vi "test_Rx Exec Unit (UDP).vi"() -> ()   [LabVIEW 2020]
uses:
  <vilib>/NI VeriStand/Custom Device API/Custom Device Item Ref.ctl
  <vilib>/NI VeriStand/Custom Device API/Custom Device API.lvlib
  Engine/Implementation/Rx UDP Execution Unit/Rx UDP Execution Unit.lvclass
  Engine/Implementation/Shared Resources/Shared Resources.lvclass
  C:/Users/Administrator/Desktop/git/niveristand-aim-arinc664-custom-device/Source/Custom Device Support/Engine/Interfaces/Shared Resources/Shared Resources.lvclass
  <instrlib>/AIM GmbH/_AIM 664/_controls/comm_verification_rx.ctl
  <instrlib>/AIM GmbH/_AIM 664/AIM664LV.lvlib
  Import/_typedefs/board_setup.ctl
  Import/AIM ARINC 664 Import.lvlib
  Shared/Encoding (Arinc664).ctl
  <instrlib>/AIM GmbH/_AIM 664/_controls/comm_udp_rx.ctl
panel:
  in  "board properties in":T1={"boardId"=1, "portSpeed"=0, "portConfig"=0} {"portConfig" items=["FDX_SINGLE", "FDX_REDUNDANT"]; "portSpeed" items=["FDX_100MBIT", "FDX_10MBIT", "FDX_AUTO_100MBIT", "FDX_AUTO_10MBIT", "FDX_AUTO_ERROR", "FDX_1000MBIT"]}
  in  "Init Shared Resources":bool
  in  "rx_param":T3(array[cluster])=[{"Data"=[0, 0, 0, 0, 0, 0, 0, 0, 0, 0, 0, 0, 0, 0, 0, 0, 0, 0, 0, 0, 0, 0, 0, 0, 0, 0, 0, 0, 0, 0, 0, 0, 0, 0, 0, 0, 0, 0, 0, 0, 0, 0, 0, 0, 0, 0, 0, 0, 0, 0, 0, 0, 0, 0, 0, 0, 0, 0, 0, 0, 0, 0, 0, 0, 0, 0, 0, 0, 0, 0, 0, 0, 0, 0, 0, 0, 0, 0, 0, 0, 0, 0, 0, 0, 0, 0, 0, 0, 0, 0, 0, 0, 0, 0, 0, 0, 0, 0, 0, 0, 0, 0, 0, 0, 0, 0, 0, 0, 0, 0, 0, 0, 0, 0, 0, 0, 0, 0, 0, 0, 0, 0, 0, 0, 0, 0, 0, 0, 0, 0, 0, 0, 0, 0, 0, 0, 0, 0, 0, 0, 0, 0, 0, 0, 0, 0, 0, 0, 0, 0, 0, 0, 0, 0, 0, 0, 0, 0, 0, 0, 0, 0, 0, 0, 0, 0, 0, 0, 0, 0, 0, 0, 0, 0, 0, 0, 0, 0, 0, 0, 0, 0, 0, 0, 0, 0, 0, 0, 0, 0, 0, 0, 0, 0, 0, 0, 0, 0, 0, 0, 0, 0, 0, 0, 0, 0, 0, 0, 0, 0, 0, 0, 0, 0, 0, 0, 0, 0, 0, 0, 0, 0, 0, 0, 0, 0, 0, 0, 0, 0, 0, 0, 0, 0, 0, 0, 0, 0, 0, 0, 0, 0, 0, 0, 0, 0, 0, 0, 0, 0, 0, 0, 0, 0, 0, 0, 0, 0, 0, 0, 0, 0, 0, 0, 0, 0, 0, 0, 0, 0, 0, 0, 0, 0, 0, 0, 0, 0, 0, 0, 0, 0, 0, 0, 0, 0, 0, 0, 0, 0, 0, 0, 0, 0, 0, 0, 0, 0, 0, 0, 0, 0, 0, 0, 0, 0, 0, 0, 0, 0, 0, 0, 0, 0, 0, 0, 0, 0, 0, 0, 0, 0, 0, 0, 0, 0, 0, 0, 0, 0, 0, 0, 0, 0, 0, 0, 0, 0, 0, 0, 0, 0, 0, 0, 0, 0, 0, 0, 0, 0, 0, 0, 0, 0, 0, 0, 0, 0, 0, 0, 0, 0, 0, 0, 0, 0, 0, 0, 0, 0, 0, 0, 0, 0, 0, 0, 0, 0, 0, 0, 0, 0, 0, 0, 0, 0, 0, 0, 0, 0, 0, 0, 0, 0, 0, 0, 0, 0, 0, 0, 0, 0, 0, 0, 0, 0, 0, 0, 0, 0, 0, 0, 0, 0, 0, 0, 0, 0, 0, 0, 0, 0, 0, 0, 0, 0, 0, 0, 0, 0, 0, 0, 0, 0, 0, 0, 0, 0, 0, 0, 0, 0, 0, 0, 0, 0, 0, 0, 0, 0, 0, 0, 0, 0, 0, 0, 0, 0, 0, 0, 0, 0, 0, 0, 0, 0, 0, 0, 0, 0, 0, 0, 0, 0, 0, 0, 0, 0, 0, 0, 0, 0, 0, 0, 0, 0, 0, 0, 0, 0, 0, 0, 0, 0, 0, 0, 0, 0, 0, 0, 0, 0, 0, 0, 0, 0, 0, 0, 0, 0, 0, 0, 0, 0, 0, 0, 0, 0, 0, 0, 0, 0, 0, 0, 0, 0, 0, 0, 0, 0, 0, 0, 0, 0, 0, 0, 0, 0, 0, 0, 0, 0, 0, 0, 0, 0, 0, 0, 0, 0, 0, 0, 0, 0, 0, 0, 0, 0, 0, 0, 0, 0, 0, 0, 0, 0, 0, 0, 0, 0, 0, 0, 0, 0, 0, 0, 0, 0, 0, 0, 0, 0, 0, 0, 0, 0, 0, 0, 0, 0, 0, 0, 0, 0, 0, 0, 0, 0, 0, 0, 0, 0, 0, 0, 0, 0, 0, 0, 0, 0, 0, 0, 0, 0, 0, 0, 0, 0, 0, 0, 0, 0, 0, 0, 0, 0, 0, 0, 0, 0, 0, 0, 0, 0, 0, 0, 0, 0, 0, 0, 0, 0, 0, 0, 0, 0, 0, 0, 0, 0, 0, 0, 0, 0, 0, 0, 0, 0, 0, 0, 0, 0, 0, 0, 0, 0, 0, 0, 0, 0, 0, 0, 0, 0, 0, 0, 0, 0, 0, 0, 0, 0, 0, 0, 0, 0, 0, 0, 0, 0, 0, 0, 0, 0, 0, 0, 0, 0, 0, 0, 0, 0, 0, 0, 0, 0, 0, 0, 0, 0, 0, 0, 0, 0, 0, 0, 0, 0, 0, 0, 0, 0, 0, 0, 0, 0, 0, 0, 0, 0, 0, 0, 0, 0, 0, 0, 0, 0, 0, 0, 0, 0, 0, 0, 0, 0, 0, 0, 0, 0, 0, 0, 0, 0, 0, 0, 0, 0, 0, 0, 0, 0, 0, 0, 0, 0, 0, 0, 0, 0, 0, 0, 0, 0, 0, 0, 0, 0, 0, 0, 0, 0, 0, 0, 0, 0, 0, 0, 0, 0, 0, 0, 0, 0, 0, 0, 0, 0, 0, 0, 0, 0, 0, 0, 0, 0, 0, 0, 0, 0, 0, 0, 0, 0, 0, 0, 0, 0, 0, 0, 0, 0, 0, 0, 0, 0, 0, 0, 0, 0, 0, 0, 0, 0, 0, 0, 0, 0, 0, 0, 0, 0, 0, 0, 0, 0, 0, 0, 0, 0, 0, 0, 0, 0, 0, 0, 0, 0, 0, 0, 0, 0, 0, 0, 0, 0, 0, 0, 0, 0, 0, 0, 0, 0, 0, 0, 0, 0, 0, 0, 0, 0, 0, 0, 0, 0, 0, 0, 0, 0, 0, 0, 0, 0, 0, 0, 0, 0, 0, 0, 0, 0, 0, 0, 0, 0, 0, 0, 0, 0, 0, 0, 0, 0, 0, 0, 0, 0, 0, 0, 0, 0, 0, 0, 0, 0, 0, 0, 0, 0, 0, 0, 0, 0, 0, 0, 0, 0, 0, 0, 0, 0, 0, 0, 0, 0, 0, 0, 0, 0, 0, 0, 0, 0, 0, 0, 0, 0, 0, 0, 0, 0, 0, 0, 0, 0, 0, 0, 0, 0, 0, 0, 0, 0, 0, 0, 0, 0, 0, 0, 0, 0, 0, 0, 0, 0, 0, 0, 0, 0, 0, 0, 0, 0, 0, 0, 0, 0, 0, 0], "Parameters"=[{"start index"=0, "size"=64, "encoding"=6, "signed"=TRUE, "scale multiplier"=1.0, "scale offset"=0.0}, {"start index"=64, "size"=64, "encoding"=6, "signed"=TRUE, "scale multiplier"=1.0, "scale offset"=0.0}, {"start index"=0, "size"=0, "encoding"=0, "signed"=FALSE, "scale multiplier"=0.0, "scale offset"=0.0}]}, {"Data"=[0, 0, 0, 0, 0, 0, 0, 0, 0, 0, 0, 0, 0, 0, 0, 0, 0, 0, 0, 0, 0, 0, 0, 0, 0, 0, 0, 0, 0, 0, 0, 0, 0, 0, 0, 0, 0, 0, 0, 0, 0, 0, 0, 0, 0, 0, 0, 0, 0, 0, 0, 0, 0, 0, 0, 0, 0, 0, 0, 0, 0, 0, 0, 0, 0, 0, 0, 0, 0, 0, 0, 0, 0, 0, 0, 0, 0, 0, 0, 0, 0, 0, 0, 0, 0, 0, 0, 0, 0, 0, 0, 0, 0, 0, 0, 0, 0, 0, 0, 0, 0, 0, 0, 0, 0, 0, 0, 0, 0, 0, 0, 0, 0, 0, 0, 0, 0, 0, 0, 0, 0, 0, 0, 0, 0, 0, 0, 0, 0, 0, 0, 0, 0, 0, 0, 0, 0, 0, 0, 0, 0, 0, 0, 0, 0, 0, 0, 0, 0, 0, 0, 0, 0, 0, 0, 0, 0, 0, 0, 0, 0, 0, 0, 0, 0, 0, 0, 0, 0, 0, 0, 0, 0, 0, 0, 0, 0, 0, 0, 0, 0, 0, 0, 0, 0, 0, 0, 0, 0, 0, 0, 0, 0, 0, 0, 0, 0, 0, 0, 0, 0, 0, 0, 0, 0, 0, 0, 0, 0, 0, 0, 0, 0, 0, 0, 0, 0, 0, 0, 0, 0, 0, 0, 0, 0, 0, 0, 0, 0, 0, 0, 0, 0, 0, 0, 0, 0, 0, 0, 0, 0, 0, 0, 0, 0, 0, 0, 0, 0, 0, 0, 0, 0, 0, 0, 0, 0, 0, 0, 0, 0, 0, 0, 0, 0, 0, 0, 0, 0, 0, 0, 0, 0, 0, 0, 0, 0, 0, 0, 0, 0, 0, 0, 0, 0, 0, 0, 0, 0, 0, 0, 0, 0, 0, 0, 0, 0, 0, 0, 0, 0, 0, 0, 0, 0, 0, 0, 0, 0, 0, 0, 0, 0, 0, 0, 0, 0, 0, 0, 0, 0, 0, 0, 0, 0, 0, 0, 0, 0, 0, 0, 0, 0, 0, 0, 0, 0, 0, 0, 0, 0, 0, 0, 0, 0, 0, 0, 0, 0, 0, 0, 0, 0, 0, 0, 0, 0, 0, 0, 0, 0, 0, 0, 0, 0, 0, 0, 0, 0, 0, 0, 0, 0, 0, 0, 0, 0, 0, 0, 0, 0, 0, 0, 0, 0, 0, 0, 0, 0, 0, 0, 0, 0, 0, 0, 0, 0, 0, 0, 0, 0, 0, 0, 0, 0, 0, 0, 0, 0, 0, 0, 0, 0, 0, 0, 0, 0, 0, 0, 0, 0, 0, 0, 0, 0, 0, 0, 0, 0, 0, 0, 0, 0, 0, 0, 0, 0, 0, 0, 0, 0, 0, 0, 0, 0, 0, 0, 0, 0, 0, 0, 0, 0, 0, 0, 0, 0, 0, 0, 0, 0, 0, 0, 0, 0, 0, 0, 0, 0, 0, 0, 0, 0, 0, 0, 0, 0, 0, 0, 0, 0, 0, 0, 0, 0, 0, 0, 0, 0, 0, 0, 0, 0, 0, 0, 0, 0, 0, 0, 0, 0, 0, 0, 0, 0, 0, 0, 0, 0, 0, 0, 0, 0, 0, 0, 0, 0, 0, 0, 0, 0, 0, 0, 0, 0, 0, 0, 0, 0, 0, 0, 0, 0, 0, 0, 0, 0, 0, 0, 0, 0, 0, 0, 0, 0, 0, 0, 0, 0, 0, 0, 0, 0, 0, 0, 0, 0, 0, 0, 0, 0, 0, 0, 0, 0, 0, 0, 0, 0, 0, 0, 0, 0, 0, 0, 0, 0, 0, 0, 0, 0, 0, 0, 0, 0, 0, 0, 0, 0, 0, 0, 0, 0, 0, 0, 0, 0, 0, 0, 0, 0, 0, 0, 0, 0, 0, 0, 0, 0, 0, 0, 0, 0, 0, 0, 0, 0, 0, 0, 0, 0, 0, 0, 0, 0, 0, 0, 0, 0, 0, 0, 0, 0, 0, 0, 0, 0, 0, 0, 0, 0, 0, 0, 0, 0, 0, 0, 0, 0, 0, 0, 0, 0, 0, 0, 0, 0, 0, 0, 0, 0, 0, 0, 0, 0, 0, 0, 0, 0, 0, 0, 0, 0, 0, 0, 0, 0, 0, 0, 0, 0, 0, 0, 0, 0, 0, 0, 0, 0, 0, 0, 0, 0, 0, 0, 0, 0, 0, 0, 0, 0, 0, 0, 0, 0, 0, 0, 0, 0, 0, 0, 0, 0, 0, 0, 0, 0, 0, 0, 0, 0, 0, 0, 0, 0, 0, 0, 0, 0, 0, 0, 0, 0, 0, 0, 0, 0, 0, 0, 0, 0, 0, 0, 0, 0, 0, 0, 0, 0, 0, 0, 0, 0, 0, 0, 0, 0, 0, 0, 0, 0, 0, 0, 0, 0, 0, 0, 0, 0, 0, 0, 0, 0, 0, 0, 0, 0, 0, 0, 0, 0, 0, 0, 0, 0, 0, 0, 0, 0, 0, 0, 0, 0, 0, 0, 0, 0, 0, 0, 0, 0, 0, 0, 0, 0, 0, 0, 0, 0, 0, 0, 0, 0, 0, 0, 0, 0, 0, 0, 0, 0, 0, 0, 0, 0, 0, 0, 0, 0, 0, 0, 0, 0, 0, 0, 0, 0, 0, 0, 0, 0, 0, 0, 0, 0, 0, 0, 0, 0, 0, 0, 0, 0, 0, 0, 0, 0, 0, 0, 0, 0, 0, 0, 0, 0, 0, 0, 0, 0, 0, 0, 0, 0, 0, 0, 0, 0, 0, 0, 0, 0, 0, 0, 0, 0, 0, 0, 0, 0, 0, 0, 0, 0, 0, 0, 0, 0, 0, 0, 0, 0, 0, 0, 0, 0, 0, 0, 0, 0, 0, 0, 0, 0, 0, 0, 0, 0, 0, 0, 0, 0, 0, 0, 0, 0, 0, 0, 0, 0, 0, 0, 0, 0, 0, 0, 0, 0, 0, 0, 0, 0, 0, 0, 0, 0, 0, 0, 0, 0, 0, 0, 0, 0, 0, 0, 0, 0, 0, 0, 0, 0, 0, 0, 0, 0, 0, 0, 0, 0, 0, 0, 0, 0, 0, 0, 0, 0, 0, 0, 0, 0, 0, 0, 0, 0, 0, 0, 0, 0, 0, 0, 0, 0, 0, 0, 0, 0, 0, 0, 0], "Parameters"=[{"start index"=0, "size"=64, "encoding"=6, "signed"=TRUE, "scale multiplier"=1.0, "scale offset"=0.0}, {"start index"=64, "size"=64, "encoding"=6, "signed"=TRUE, "scale multiplier"=1.0, "scale offset"=0.0}, {"start index"=0, "size"=0, "encoding"=0, "signed"=FALSE, "scale multiplier"=0.0, "scale offset"=0.0}]}] {"Parameters"."encoding" items=["BNR", "BCD", "Discrete"]}
  in  "VL Configurations":T6(array[cluster])=[{"VL Config"={"VlId"=60, "VLRange"=1, "VerificationMode"=0, "Bag"=0, "Jitter"=0, "MaxFrameLength"=0, "MaxSkew"=0, "VLBufSize"=32768, "FilterMode"=0, "FilterPosition"=0, "Padding"=0, "FilterMask"=0, "FilterData"=0, "MinFrameLength"=0}, "CommPort Config"=[{"PortType"=enum."FDX_UDP_SAMPLING", "SubVIId"=0, "domainID"=1, "sideID"=1, "locationID"=1, "partitionID"=1, "UdpSrcPort"=24, "UdpDstPort"=23, "UdpNumBufMessages"=1, "UdpMaxMessageSize"=512, "UdpSamplingRate"=0}, {"PortType"=enum."FDX_UDP_SAMPLING", "SubVIId"=0, "domainID"=2, "sideID"=1, "locationID"=1, "partitionID"=1, "UdpSrcPort"=34, "UdpDstPort"=33, "UdpNumBufMessages"=1, "UdpMaxMessageSize"=512, "UdpSamplingRate"=0}]}] {"VL Config"."FilterMode" items=["FDX_RX_VL_FLT_DIS", "FDX_RX_VL_FLT_ENA ", "FDX_RX_VL_FLT_ENA_INV"]; "VL Config"."VLBufSize" format="%.0x"; "VL Config"."VerificationMode" items=["FDX_RX_VL_CHECK_ENA_DEFAULT"=65535, "FDX_RX_VL_CHECK_REDMAM"=16, "DX_RX_VL_CHECK_TRAFIC"=8, "FDX_RX_VL_CHECK_FRAMESIZE"=4, "FDX_RX_VL_CHECK_SNINTEG"=2, "FDX_RX_VL_CHECK_INVPAC"=1, "FDX_RX_VL_CHECK_DISA"=0]}
  in  "port id":u32
  in  "board id":u32=1
  out "exec time us":u32(graph)=2
  out "Values out":dbl[](array[numeric])
  out "error out":errorcluster
  in  "stop":bool
  in  "loop rate mS":u32=10
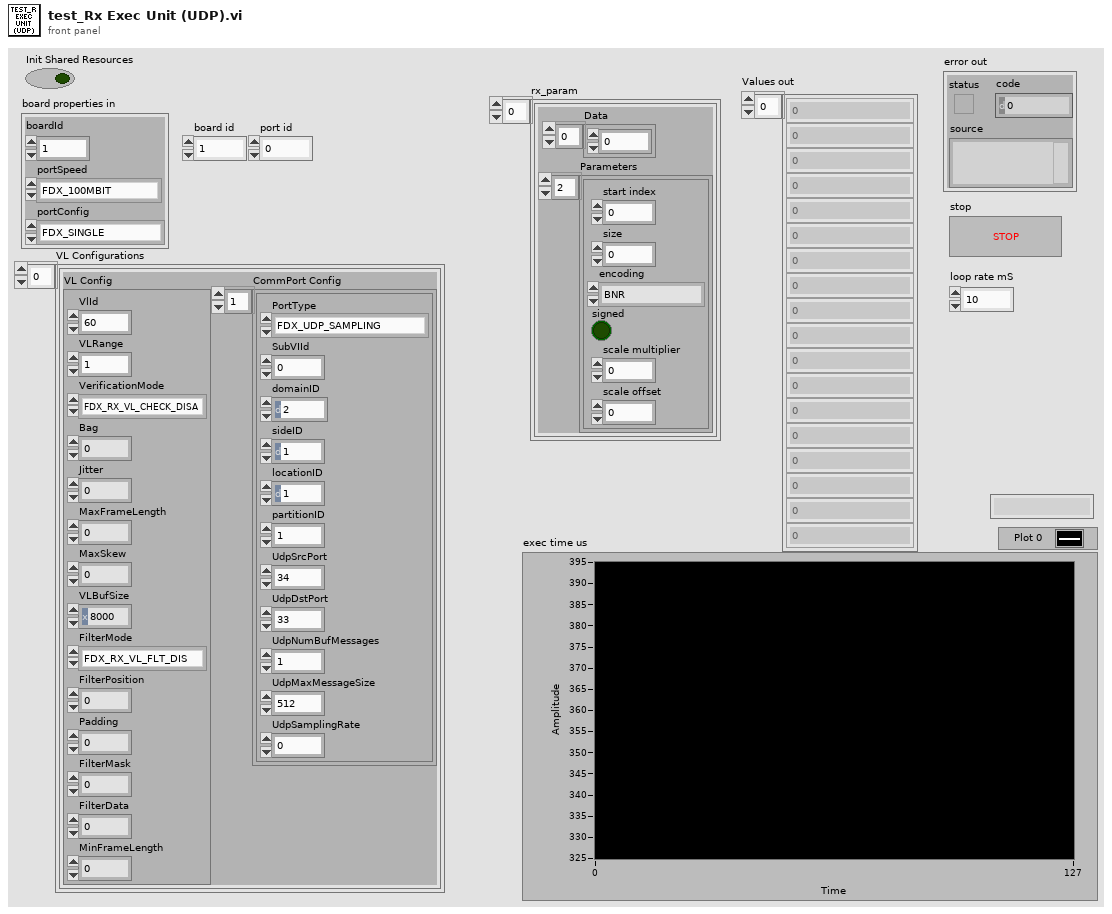
[diagram p1: front panel]
types:
  T1 = typedef "AIM ARINC 664 Import.lvlib/board_setup.ctl" = cluster{"boardId":u32, "portSpeed":u32, "portConfig":u32}
  T2 = typedef "Encoding (Arinc664).ctl" = u16
  T3 = cluster{"Data":u8[], "Parameters":cluster{"start index":i32, "size":i32, "encoding":T2, "signed":bool, "scale multiplier":dbl, "scale offset":dbl}[]}[]
  T4 = typedef "AIM664LV.lvlib/comm_verification_rx.ctl" = cluster{"VlId":u16, "VLRange":u32, "VerificationMode":u32, "Bag":u32, "Jitter":u32, "MaxFrameLength":u32, "MaxSkew":u32, "VLBufSize":u32, "FilterMode":u32, "FilterPosition":u32, "Padding":u32, "FilterMask":u32, "FilterData":u32, "MinFrameLength":u32}
  T5 = typedef "AIM664LV.lvlib/comm_udp_rx.ctl" = cluster{"PortType":enum16{"FDX_UDP_SAMPLING", "FDX_UDP_QUEUING"}, "SubVIId":u32, "domainID":u8, "sideID":u8, "locationID":u8, "partitionID":u8, "UdpSrcPort":u16, "UdpDstPort":u16, "UdpNumBufMessages":u32, "UdpMaxMessageSize":u32, "UdpSamplingRate":u32}
  T6 = cluster{"VL Config":T4, "CommPort Config":T5[]}[]
  T7 = typedef "Custom Device API.lvlib/Custom Device Item Ref.ctl" = u64
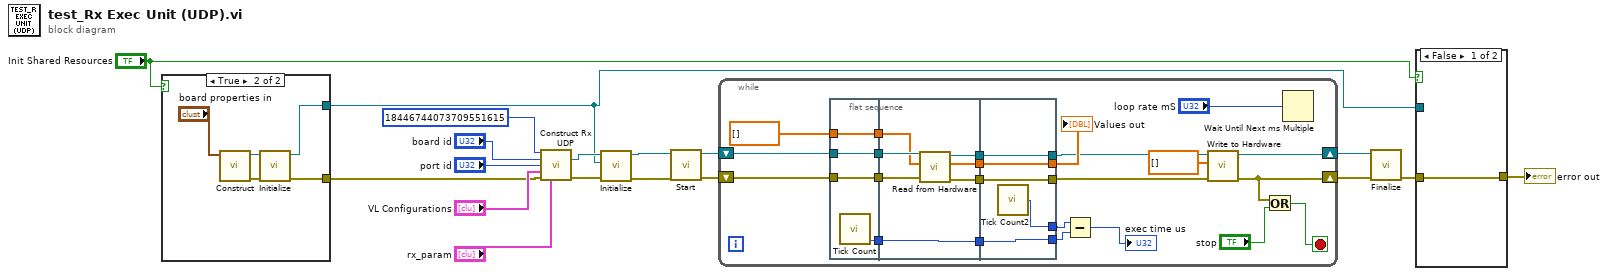
[diagram p0: block diagram]
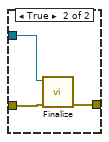
[diagram p2: hidden frame]
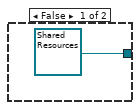
[diagram p3: hidden frame]
diagram:
  n1 = case shown="True" "Init Shared Resources" {
    tunnel: [refnum<class "Shared Resources.lvclass"> refnum ("Shared Resources out") w22] -> w1
    tunnel: [_ w21] -> w5
    frame False {
    }
    frame True {
      n2 = call "Construct.vi"("board properties in"="board properties in") -> ("error out"=w23:errorcluster, "Shared Resources out"=w24:refnum<class "Shared Resources.lvclass">)  [unwired: 9 in]
      n3 = call-dynamic "Initialize.vi"("error in"=w23, "Shared Resources in"=w24) -> ("error out"=w21:errorcluster, "Shared Resources out"=w22:refnum<class "Shared Resources.lvclass">)  [unwired: 8 in]
    }
  }
  n4 = call "Construct Rx UDP.vi"("custom device ref in"=T7 18446744073709551615, "InstrumentHandle_board"="board id", "InstrumentHandle_port"="port id", "VL Configurations"="VL Configurations", "error in (no error)"=w5, "CommPort Payload"="rx_param") -> ("Execution Unit Out"=w11:refnum<class "Rx UDP Execution Unit.lvclass">, "error out"=w12:errorcluster)  [unwired: 7 in, 1 out]
  n5 = call-dynamic "Initialize.vi"("error in"=w12, "shared resources"=w1, "Rx UDP Execution Unit in"=w11) -> ("error out"=w13:errorcluster, "Rx UDP Execution Unit out"=w18:refnum<class "Rx UDP Execution Unit.lvclass">)  [unwired: 7 in]
  n6 = call-dynamic "Start.vi"("error in"=w13, "Rx UDP Execution Unit in"=w18) -> ("error out"=w16:errorcluster, "Rx UDP Execution Unit out"=w17:refnum<class "Rx UDP Execution Unit.lvclass">)  [unwired: 8 in]
  n7 = while {
    shift-right: [w27] -> w15
    shift-left: w17 -> [w47]
    shift-right: [w26] -> w14
    shift-left: w16 -> [w46]
    stop <- w43 stop-if-true
    n8 = flat-sequence {
      tunnel: dbl[] [] ("Values in") -> [w49]
      tunnel: w46 -> [w50]
      tunnel: w47 -> [w51]
      tunnel: [w51] -> w37
      tunnel: [w50] -> w36
      tunnel: [w49] -> w35
      tunnel: [w48] -> w33
      tunnel: [w56] -> w40
      tunnel: [w55] -> w39
      tunnel: [w54] -> w38
      tunnel: w37 -> [w58]
      tunnel: w36 -> [w57]
      tunnel: w35 -> [w53]
      tunnel: [w52] -> w34
      tunnel: w33 -> [w52]
      tunnel: [w61] -> w42
      tunnel: [w62] -> w28
      tunnel: [w63] -> w29
      tunnel: w40 -> [w63]
      tunnel: w39 -> [w62]
      tunnel: w38 -> [w61]
      tunnel: [w60] -> w32
      tunnel: w34 -> [w60]
      tunnel: [w59] -> w31
      frame #0 {
        n9 = call "Tick Count"() -> ("Tick Count(uSec)"=w48:u32)
      }
      frame #1 {
        n10 = call-dynamic "Read from Hardware.vi"("error in"=w57, "Values in"=w53, "Rx UDP Execution Unit in"=w58) -> ("error out"=w55:errorcluster, "Values out"=w54:dbl[], "Rx UDP Execution Unit out"=w56:refnum<class "Rx UDP Execution Unit.lvclass">)  [unwired: 6 in]
      }
      frame #2 {
        n11 = call "Tick Count2"() -> ("Tick Count(uSec)"=w59:u32)
      }
    }
    n12 = Subtract(x=w31, y=w32) -> (x-y=→"exec time us":u32)
    n13 = call-dynamic "Write to Hardware.vi"("error in"=w28, "Values in"=dbl[] [], "Rx UDP Execution Unit in"=w29) -> ("error out"=w26:errorcluster, "Rx UDP Execution Unit out"=w27:refnum<class "Rx UDP Execution Unit.lvclass">)  [unwired: 5 in, 2 out]
    n14 = Or(x=w26, y="stop") -> (x .or. y?=w43:bool)
    n15 = Wait Until Next ms Multiple(millisecond multiple="loop rate mS") -> ()  [unwired: 1 out]
    "Values out" <- w42
  }
  n16 = call-dynamic "Finalize.vi"("error in"=w14, "Rx UDP Execution Unit in"=w15) -> ("error out"=w3:errorcluster)  [unwired: 8 in, 1 out]
  n17 = case shown="False" "Init Shared Resources" {
    tunnel: w3 -> [w64 w66]
    tunnel: [w64 w67] -> w2
    tunnel: w1 -> [_ w65]
    frame False {
    }
    frame True {
      n18 = call-dynamic "Finalize.vi"("error in"=w66, "Shared Resources in"=w65) -> ("error out"=w67:errorcluster)  [unwired: 8 in, 1 out]
    }
  }
  "error out" <- w2
